vi "Get Wall Clock Time.vi"() -> (5 "Time (ns)":i64)   [LabVIEW 2021, in "Time_CIF_U.lvlib"]
doc: "Wall clock is defined as the OS time as it appears in human facing UI elements. It is the basis for some system functions such as syslog."
uses:
  Time_CIF_U.lvlib
  Typedef/Linux Timestruct.ctl
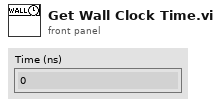
[diagram p1: front panel]
types:
  T1 = typedef "Time_CIF_U.lvlib/Linux Timestruct.ctl" = cluster{"tm_sec":i32, "tm_min":i32, "tm_hour":i32, "tm_mday":i32, "tm_mon":i32, "tm_year":i32, "tm_wday":i32, "tm_yday":i32, "tm_isdst":i32, "padding":i32, "tm_gmtoff":i64, "tm_zone_ptr":i64, "end pad":i64}
  T2 = typedef "LVDateTimeRec.ctl" = cluster{"fractional second":dbl, "second":i32, "minute":i32, "hour":i32, "day of month":i32, "month":i32, "year":i32, "day of week":i32, "day of year":i32, "DST":i32}
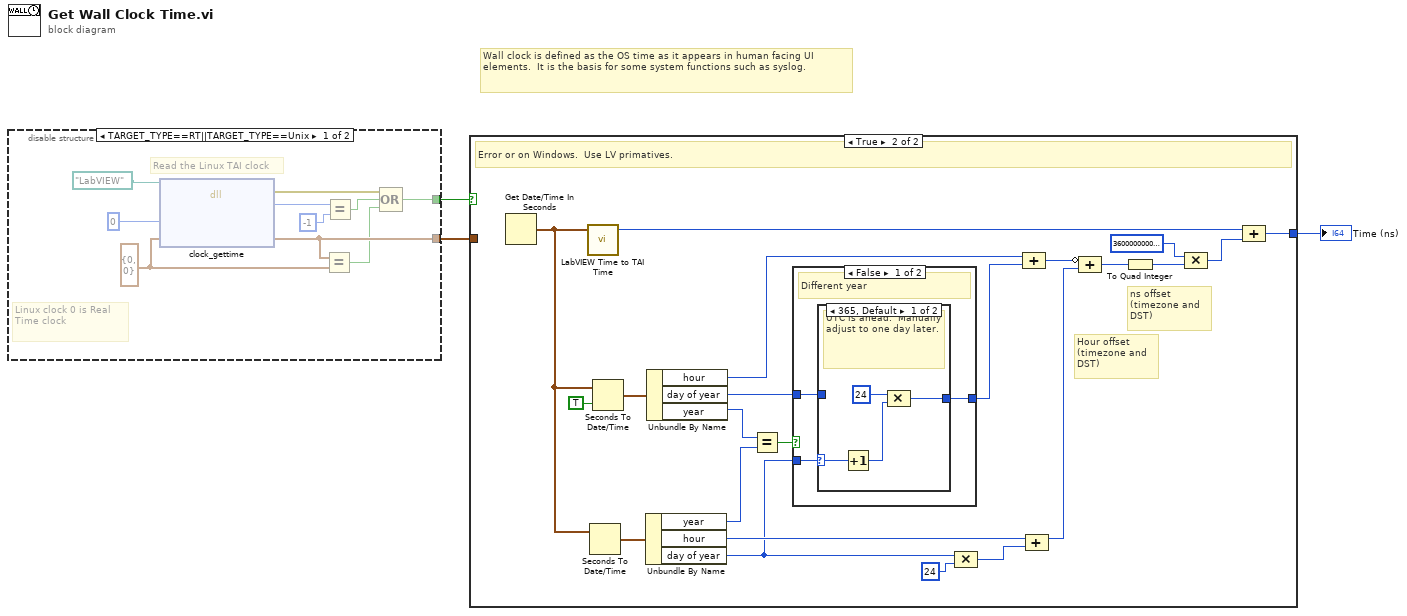
[diagram p0: block diagram]
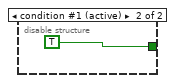
[diagram p2: hidden frame]
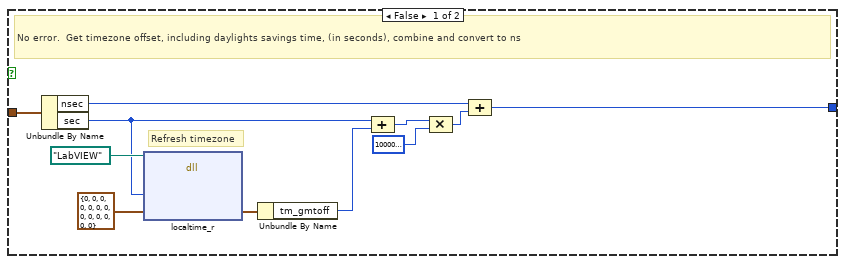
[diagram p3: hidden frame]
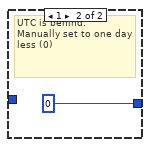
[diagram p4: hidden frame]
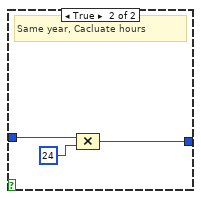
[diagram p5: hidden frame]
diagram:
  # "Wall clock is defined as the OS time as it appears in human facing UI elements.  It is the basis for some system functions such as syslog."
  n1 = disable-structure shown="TARGET_TYPE==RT||TARGET_TYPE==Unix" {
    disable-tunnel: [w8 TRUE] -> w1
    disable-tunnel: [w6 _] -> w2
    frame condition #0 {
      w5 = cluster{"sec":i64, "nsec":i64} {"sec"=0, "nsec"=0} ("timespec")
      # "Read the Linux TAI clock"
      # "Linux clock 0 is Real Time clock"
      n2 = dll-call lib="lib/libc.so.6" fn="clock_gettime"(path in=path "LabVIEW" ("Path"), "clock_id"=u32 0, "timespec"=w5) -> (error out=w9:errorcluster, "status"=w13:i32, "timespec"=w6:cluster{"sec":i64, "nsec":i64})  [unwired: 3 in, 1 out]
      n3 = Equal?(x=w6, y=w5) -> (x = y?=w4:bool)
      n4 = Equal?(x=w13, y=-1) -> (x = y?=w10:bool)
      n5 = Compound Arithmetic op=OR(w9, w10, w4) -> (w8:bool)
    }
    frame condition #1 (active) {
    }
  }
  n6 = case shown="True" w1 {
    tunnel: w2 -> [w24 _]
    tunnel: [w21 w26] -> w3
    frame False {
      # "Refresh timezone"
      # "No error.  Get timezone offset, including daylights savings time, (in seconds), combine and convert to ns"
      n7 = Unbundle By Name(w24) -> ("nsec"=w23:i64, "sec"=w18:i64)
      n8 = dll-call lib="lib/libc.so.6" fn="localtime_r"(path in=path "LabVIEW" ("Path"), "timer"=w18, "time_struct"=T1 {"tm_sec"=0, "tm_min"=0, "tm_hour"=0, "tm_mday"=0, "tm_mon"=0, "tm_year"=0, "tm_wday"=0, "tm_yday"=0, "tm_isdst"=0, "padding"=0, "tm_gmtoff"=0, "tm_zone_ptr"=0, "end pad"=0}) -> ("time_struct"=w16:T1)  [unwired: 4 in, 2 out]
      n9 = Unbundle By Name(w16) -> ("tm_gmtoff"=w15:i64)
      n10 = Compound Arithmetic op=ADD(w18, w15) -> (w17:i64)
      n11 = Compound Arithmetic op=MULTIPLY(w17, i64 1000000000 ("x")) -> (w22:i64)
      n12 = Compound Arithmetic op=ADD(w23, w22) -> (w21:i64)
    }
    frame True {
      # "ns offset (timezone and DST)"
      # "Hour offset (timezone and DST)"
      # "Error or on Windows.  Use LV primatives."
      n13 = Get Date/Time In Seconds() -> (seconds since 1Jan1904=w47:timestamp)
      n14 = call "LabVIEW Time to TAI Time.vi"("LabVIEW Time (s)"=w47) -> ("TAI Time (ns)"=w31:i64)  [unwired: 4 in]
      n15 = Seconds To Date/Time(time stamp (now)=w47) -> (date time rec=w44:T2)  [unwired: 1 in]
      n16 = Seconds To Date/Time(time stamp (now)=w47, to UTC (F)=TRUE) -> (date time rec=w45:T2)
      n17 = Unbundle By Name(w44) -> ("year"=w36:i32, "hour"=w35:i32, "day of year"=w34:i32)
      n18 = Unbundle By Name(w45) -> ("hour"=w42:i32, "day of year"=w43:i32, "year"=w37:i32)
      n19 = Equal?(x=w37, y=w36) -> (x = y?=w38:bool)
      n20 = case shown="False" w38 {
        tunnel: w43 -> [w50 w58]
        tunnel: [w49 w56] -> w39
        tunnel: w34 -> [w48 _]
        frame False {
          # "Different year"
          n21 = case shown="365, Default" w48 {
            selector: w48 -> [w51 _]
            tunnel: w50 -> [_ _]
            tunnel: [w52 0] -> w49
            frame 365, Default {
              # "UTC is ahead.  Manually adjust to one day later."
              n22 = Increment(x=w51) -> (x+1=w54:i32)
              n23 = Compound Arithmetic op=MULTIPLY(24 ("value"), w54) -> (w52:i32)
            }
            frame 1 {
              # "UTC is behind.  Manually set to one day less (0)"
            }
          }
        }
        frame True {
          # "Same year, Cacluate hours"
          n24 = Compound Arithmetic op=MULTIPLY(w58, 24 ("value")) -> (w56:i32)
        }
      }
      n25 = Compound Arithmetic op=MULTIPLY(w34, 24 ("value")) -> (w40:i32)
      n26 = Compound Arithmetic op=ADD(w42, w39) -> (w32:i32)
      n27 = Compound Arithmetic op=ADD(w35, w40) -> (w33:i32)
      n28 = Compound Arithmetic op=ADD(invert w32, w33) -> (w30:i32)
      n29 = To Quad Integer(1:w30) -> (0:w29:i64)
      n30 = Compound Arithmetic op=MULTIPLY(i64 3600000000000 ("value"), w29) -> (w27:i64)
      n31 = Compound Arithmetic op=ADD(w31, w27) -> (w26:i64)
    }
  }
  "Time (ns)" <- w3
